vi "Main Page.vi"(8 "error in (no error)":errorcluster, 11 "Node Ptr":T1 format="%.0x") -> (0 "error out":errorcluster)   [LabVIEW 2019, in "RMXVisaControl System Explorer.lvlib"]
uses:
  RMXVisaControl System Explorer.lvlib
  <vilib>/NI VeriStand/Custom Device API/Custom Device Item Ref.ctl
  Shared/Constants.vi
  <vilib>/NI VeriStand/Custom Device API/Get Item Property (I32).vi
  <vilib>/NI VeriStand/Custom Device API/Get Item Property (String).vi
  <vilib>/NI VeriStand/Custom Device API/Set Item Property (String).vi
  <vilib>/NI VeriStand/Custom Device API/Set Item Property (I32).vi
  <vilib>/NI VeriStand/Custom Device API/Custom Device API.lvlib
  Shared/RMXVisaControl Shared.lvlib
panel:
  in  "Help Ring":u16(ring)
  in  "Help":bool
  in  "Operation Mode":i32(ring) items=["Constant Current", "Constant Voltage"]
  in  "VISA resource name":refnum<visa-resource-name>
  in  "Header":cluster{"Section Name":string}={"Section Name"="Custom Device Item Settings"}
  in  "Description":string
  in  "Name":string
  # "Example: TCPIP0::10.116.1.98::hislip0::INSTR"
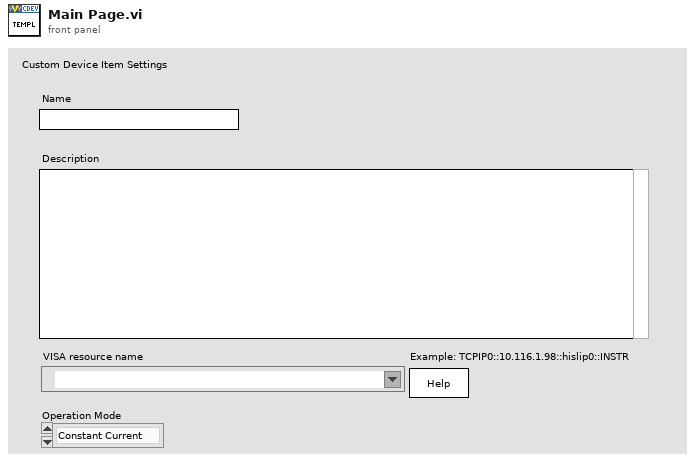
[diagram p1: front panel]
types:
  T1 = typedef "Custom Device API.lvlib/Custom Device Item Ref.ctl" = u64
  T2 = typedef "Custom Device API.lvlib/Custom Device Item Info.ctl" = cluster{"Name":string, "Is Channel":bool, "GUID":string, "Is Waveform":bool}
  T3 = typedef "Custom Device API.lvlib/Custom Device Commands.ctl" = enum16{"Default", "Item renamed", "Shutdown", "Dynamic button pressed"}
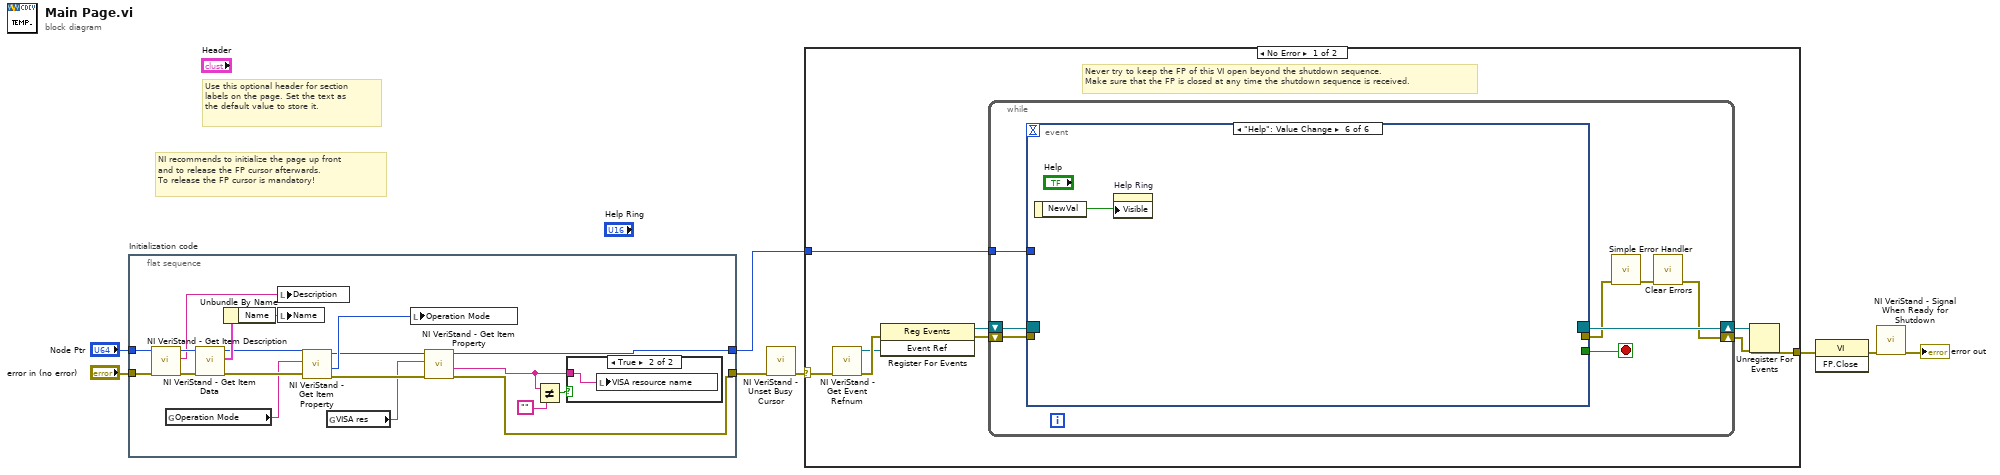
[diagram p0: block diagram]
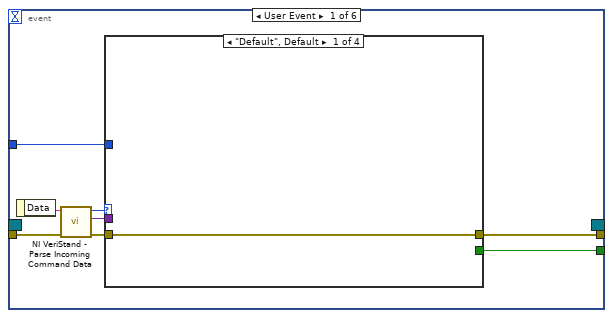
[diagram p2: hidden frame]
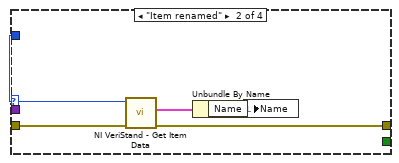
[diagram p3: hidden frame]
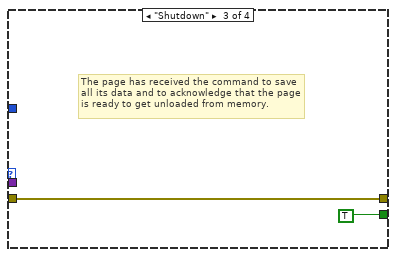
[diagram p4: hidden frame]
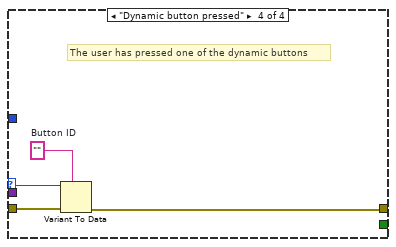
[diagram p5: hidden frame]
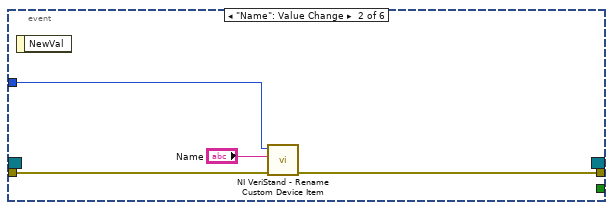
[diagram p6: hidden frame]
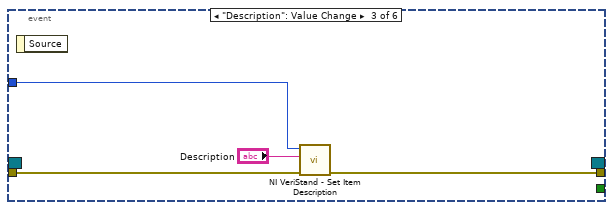
[diagram p7: hidden frame]
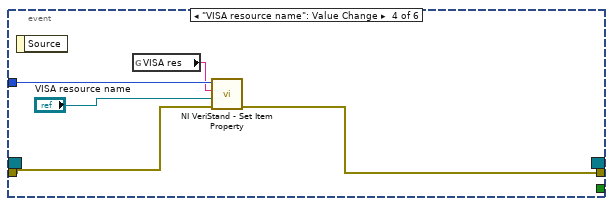
[diagram p8: hidden frame]
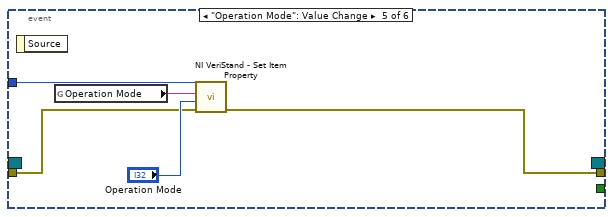
[diagram p9: hidden frame]
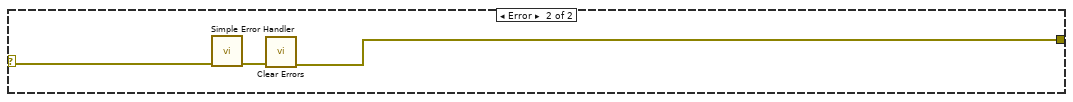
[diagram p10: hidden frame]
diagram:
  # "Use this optional header for section labels on the page. Set the text as the default value to store it."
  # "NI recommends to initialize the page up front\nand to release the FP cursor afterwards.\nTo release the FP cursor is mandatory!"
  n1 = flat-sequence "Initialization code" {
    tunnel: "error in (no error)" -> [w26]
    tunnel: "Node Ptr" -> [w25]
    tunnel: [w12] -> w4
    tunnel: [w18] -> w1
    frame #0 {
      n2 = call <vilib>:"NI VeriStand - Get Item Description.vi"("error in (no error)"=w26, "Item Ref in"=w25) -> ("error out"=w23:errorcluster, "Description"=w24:string, "Item Ref out"=w27:T1)  [unwired: 7 out]
      n3 = global read "Constants.vi" "Operation Mode"() -> (w17:string)
      n4 = call <vilib>:"NI VeriStand - Get Item Data.vi"("error in (no error)"=w23, "Item Ref in"=w27) -> ("error out"=w19:errorcluster, "Item Info"=w22:T2, "Item Ref out"=w20:T1)  [unwired: 7 out]
      n5 = Unbundle By Name(w22) -> ("Name"=w21:string)
      n6 = local write "Description"(w24) -> ()
      n7 = local write "Name"(w21) -> ()
      n8 = call-poly <vilib>:"NI VeriStand - Get Item Property.vi"("error in (no error)"=w19, "Property Name"=w17, "Item Ref in"=w20) -> ("error out"=w15:errorcluster, "Value"=w16:i32, "Item Ref out"=w14:T1)  [unwired: 5 in, 1 out]
      n9 = global read "Constants.vi" "VISA res"() -> (w13:string)
      n10 = local write "Operation Mode"(w16) -> ()
      n11 = call-poly <vilib>:"NI VeriStand - Get Item Property.vi"("error in (no error)"=w15, "Property Name"=w13, "Item Ref in"=w14) -> ("error out"=w12:errorcluster, "Value"=w10:string, "Item Ref out"=w18:T1)  [unwired: 5 in, 1 out]
      n12 = Not Equal?(x=w10, y="") -> (x != y?=w11:bool)
      n13 = case shown="True" w11 {
        tunnel: w10 -> [_ w28]
        frame False {
        }
        frame True {
          n14 = local write "VISA resource name"(w28) -> ()
        }
      }
    }
  }
  n15 = call <vilib>:"NI VeriStand - Unset Busy Cursor.vi"("error in (no error)"=w4) -> ("error out"=w3:errorcluster)  [unwired: 10 out]
  n16 = case shown="No Error" w3 {
    selector: w3 -> [w29 w87]
    tunnel: [w34 w85] -> w8
    tunnel: w1 -> [w30 _]
    frame No Error {
      # "Never try to keep the FP of this VI open beyond the shutdown sequence.\nMake sure that the FP is closed at any time the shutdown sequence is received."
      n17 = call <vilib>:"NI VeriStand - Get Event Refnum.vi"("error in (no error)"=w29) -> ("error out"=w37:errorcluster, "Event Ref"=w33:refnum<user-event>)  [unwired: 9 out]
      n18 = register-events(error in=w37, w33) -> (reference out=w31:refnum<event-registration>, error out=w32:errorcluster)  [unwired: 1 in]
      n19 = while {
        tunnel: w30 -> [w41]
        shift-right: [w38] -> w35
        shift-left: w32 -> [w44]
        shift-right: [w45] -> w36
        shift-left: w31 -> [w43]
        stop <- w42 stop-if-true
        n20 = event shown="[5] \"Help\": Value Change" {
          selector: w43 -> [_ _ _ _ _ _]
          dyn-events: [_ _ _ _ _ _] -> w45
          timeout: _ -> [_ _ _ _ _ _]
          tunnel: w44 -> [w53 w69 w72 w74 w80 _]
          tunnel: [w49 _ _ _ _ _] -> w42
          tunnel: [w48 w68 w71 w76 w79 _] -> w40
          tunnel: w41 -> [w47 w67 w73 w78 w81 _]
          event User Event {
            n21 = event-data() -> ("Data"=w52:string)  [unwired: 1 out]
            n22 = call <vilib>:"NI VeriStand - Parse Incoming Command Data.vi"("error in (no error)"=w53, "Incoming data"=w52) -> ("error out"=w51:errorcluster, "Outgoing data"=w46:variant, "Action"=w50:T3)  [unwired: 7 out]
            n23 = case shown="\"Default\", Default" w50 {
              tunnel: w51 -> [w54 w59 w60 w65]
              tunnel: [_ _ TRUE _] -> w49
              tunnel: [w54 w56 w60 w62] -> w48
              tunnel: w47 -> [_ w58 _ _]
              tunnel: w46 -> [_ _ _ w64]
              frame "Default", Default {
              }
              frame "Item renamed" {
                n24 = call <vilib>:"NI VeriStand - Get Item Data.vi"("error in (no error)"=w59, "Item Ref in"=w58) -> ("error out"=w56:errorcluster, "Item Info"=w57:T2)  [unwired: 8 out]
                n25 = Unbundle By Name(w57) -> ("Name"=w55:string)
                n26 = local write "Name"(w55) -> ()
              }
              frame "Shutdown" {
                # "The page has received the command to save all its data and to acknowledge that the page is ready to get unloaded from memory."
              }
              frame "Dynamic button pressed" {
                w63 = ""  # Button ID
                # "The user has pressed one of the dynamic buttons"
                n27 = Variant To Data(error in=w65, type=w63, Variant=w64) -> (error out=w62:errorcluster)  [unwired: 1 out]
              }
            }
          }
          event "Name": Value Change {
            n28 = event-data() -> ()  [unwired: 2 out]
            n29 = call <vilib>:"NI VeriStand - Rename Custom Device Item.vi"("error in (no error)"=w69, "New Name"="Name", "Item Ref in"=w67) -> ("error out"=w68:errorcluster)  [unwired: 1 in, 7 out]
          }
          event "Description": Value Change {
            n30 = event-data() -> ()  [unwired: 2 out]
            n31 = call <vilib>:"NI VeriStand - Set Item Description.vi"("error in (no error)"=w72, "Description"="Description", "Item Ref in"=w73) -> ("error out"=w71:errorcluster)  [unwired: 8 out]
          }
          event "VISA resource name": Value Change {
            n32 = event-data() -> ()  [unwired: 2 out]
            n33 = global read "Constants.vi" "VISA res"() -> (w77:string)
            n34 = call-poly <vilib>:"NI VeriStand - Set Item Property.vi"("error in (no error)"=w74, "Value"="VISA resource name", "Property Name"=w77, "Item Ref in"=w78) -> ("error out"=w76:errorcluster)  [unwired: 5 in, 2 out]
          }
          event "Operation Mode": Value Change {
            n35 = event-data() -> ()  [unwired: 2 out]
            n36 = global read "Constants.vi" "Operation Mode"() -> (w82:string)
            n37 = call-poly <vilib>:"NI VeriStand - Set Item Property.vi"("error in (no error)"=w80, "Value"="Operation Mode", "Property Name"=w82, "Item Ref in"=w81) -> ("error out"=w79:errorcluster)  [unwired: 5 in, 2 out]
          }
          event "Help": Value Change {
            n38 = event-data() -> ("NewVal"=w84:bool)  [unwired: 1 out]
            n39 = property on="Help Ring" class="Ring (strict)"("Visible"=w84) -> ()  [unwired: 2 in, 2 out]
          }
        }
        n40 = call <vilib>:"Simple Error Handler.vi"("error in (no error)"=w40) -> ("error out"=w39:errorcluster)  [unwired: 1 in, 7 out]
        n41 = call <vilib>:"Clear Errors.vi"("error in (no error)"=w39) -> ("error out"=w38:errorcluster)  [unwired: 1 in, 5 out]
      }
      n42 = Unregister For Events(event registration refnum=w36, error in=w35) -> (error out=w34:errorcluster)
    }
    frame Error {
      n43 = call <vilib>:"Simple Error Handler.vi"("error in (no error)"=w87) -> ("error out"=w86:errorcluster)  [unwired: 1 in, 7 out]
      n44 = call <vilib>:"Clear Errors.vi"("error in (no error)"=w86) -> ("error out"=w85:errorcluster)  [unwired: 1 in, 5 out]
    }
  }
  n45 = invoke class="VI" method="FP.Close"(error in=w8) -> (error out=w7:errorcluster)  [unwired: 2 in, 2 out]
  n46 = call <vilib>:"NI VeriStand - Signal When Ready for Shutdown.vi"("error in (no error)"=w7) -> ("error out"=→"error out":errorcluster)  [unwired: 10 out]
